vi "1 Tap 42-Bit RGB.vi"() -> ()   [LabVIEW 2014]
uses:
  <vilib>/rvi/eio/common/nirviEmuTemplateMethod_errors.vi
  <vilib>/eio/EIONode/EIONode.xnode
panel:
  out "PixelData":u64
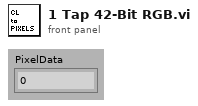
[diagram p1: front panel]
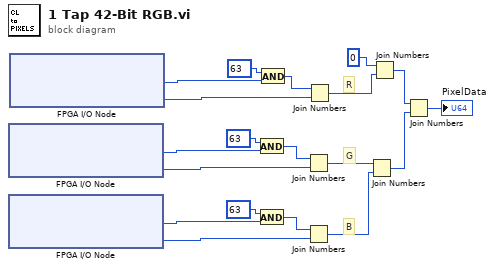
[diagram p0: block diagram]
diagram:
  # "B"
  # "R"
  # "G"
  n1 = xnode "FPGA I/O Node"() -> ("IO Module\\CL Port E"=w6:u8, "IO Module\\CL Port D"=w7:u8)  [unwired: 2 in, 2 out]
  n2 = xnode "FPGA I/O Node"() -> ("IO Module\\CL Port F"=w5:u8, "IO Module\\CL Port C"=w4:u8)  [unwired: 2 in, 2 out]
  n3 = xnode "FPGA I/O Node"() -> ("IO Module\\CL Port B"=w11:u8, "IO Module\\CL Port A"=w17:u8)  [unwired: 2 in, 2 out]
  n4 = And(x=u8 63 ("hi"), y=w6) -> (x .and. y?=w16:u8)
  n5 = And(x=u8 63 ("hi"), y=w5) -> (x .and. y?=w2:u8)
  n6 = And(x=u8 63 ("hi"), y=w11) -> (x .and. y?=w18:u8)
  n7 = Join Numbers(hi=w16, lo=w7) -> ((hi.lo)=w13:u16)
  n8 = Join Numbers(hi=w2, lo=w4) -> ((hi.lo)=w1:u16)
  n9 = Join Numbers(hi=w18, lo=w17) -> ((hi.lo)=w14:u16)
  n10 = Join Numbers(hi=w13, lo=w1) -> ((hi.lo)=w8:u32)
  n11 = Join Numbers(hi=u16 0, lo=w14) -> ((hi.lo)=w10:u32)
  n12 = Join Numbers(hi=w10, lo=w8) -> ((hi.lo)=→"PixelData":u64)
